vi "Get Weight.vi"(8 "error in (no error)":errorcluster caption="entrée d'erreur (pas d'erreur)", 11 "Class Balance_Adam_GBK en entrée":refnum<class "Class Balance_Adam_GBK.lvclass">) -> (0 "error out":errorcluster caption="sortie d'erreur", 2 "Get Weight":dbl, 3 "Class Balance_Adam_GBK en sortie":refnum<class "Class Balance_Adam_GBK.lvclass">)   [LabVIEW 2020, in "Library Instrument & Equipement.lvlib" / "Library Balance.lvlib" / "Class Balance_Adam_GBK.lvclass"]
uses:
  Class Balance_Adam_GBK.lvclass
  C:/Users/ngarcin/OneDrive - Altyor/Standard TB/Class/Balance/Balance (Default)/Class Balance (Default).lvclass
  Class Balance_Adam_GBK.lvclass/Class Balance_Adam_GBK.ctl
  Commun VI/Library Commun.lvlib
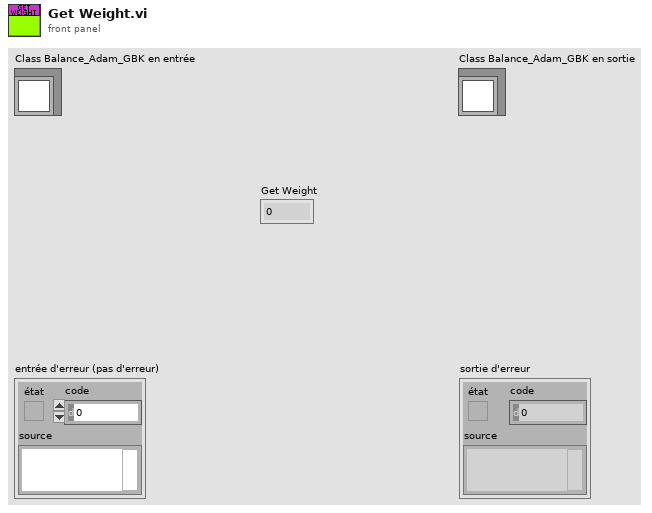
[diagram p1: front panel]
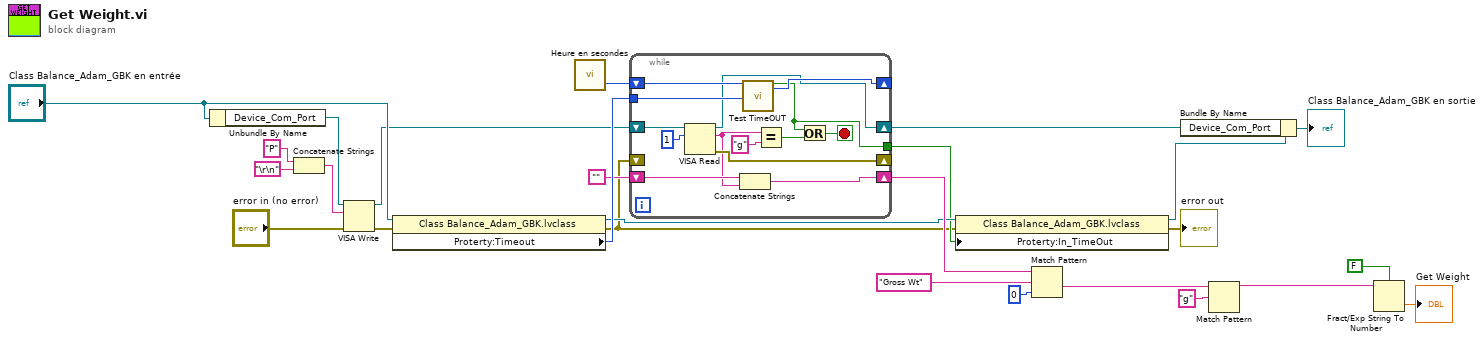
[diagram p0: block diagram]
diagram:
  n1 = Unbundle By Name("Class Balance_Adam_GBK en entrée") -> ("Device_Com_Port"=w22:refnum<visa-resource-name>)
  n2 = Concatenate Strings("P" ("chaîne"), "\r\n") -> (w25:string)
  n3 = VISA Write(VISA resource name=w22, write buffer=w25, error in (no error)="error in (no error)") -> (VISA resource name out=w17:refnum<visa-resource-name>, error out=w20:errorcluster)  [unwired: 1 out]
  n4 = property class="Class Balance_Adam_GBK.lvclass"(reference="Class Balance_Adam_GBK en entrée", error in=w20) -> (reference out=w5:refnum<class "Class Balance_Adam_GBK.lvclass">, error out=w1:errorcluster, "Proterty:Timeout"=w18:u32)
  n5 = call "Heure en secondes.vi"() -> ("Heure en milisecondes"=w21:u32)  [unwired: 2 in, 1 out]
  n6 = while {
    shift-right: [w39] -> _
    shift-left: w21 -> [w40]
    tunnel: w18 -> [w38]
    shift-right: [w34] -> w8
    shift-left: "" -> [w35]
    shift-right: [w33] -> _
    shift-left: w1 -> [_]
    shift-right: [w29] -> w15
    shift-left: w17 -> [w37]
    tunnel: [w27] -> w4
    stop <- w28 stop-if-true
    n7 = VISA Read(VISA resource name=w37, byte count=u32 1 ("nombre d'octets")) -> (VISA resource name out=w29:refnum<visa-resource-name>, read buffer=w32:string, error out=w33:errorcluster)  [unwired: 1 in, 1 out]
    n8 = Concatenate Strings(w35, w32) -> (w34:string)
    n9 = call "Test TimeOUT.vi"("OLD Time"=w40, "TimeOut ms"=w38) -> ("Timeout ?"=w27:bool, "NEW Time"=w39:u32)  [unwired: 13 in, 3 out]
    n10 = Equal?(x=w32, y="g") -> (x = y?=w30:bool)
    n11 = Or(x=w27, y=w30) -> (x .or. y?=w28:bool)
  }
  n12 = property class="Class Balance_Adam_GBK.lvclass"(reference=w5, error in=w1, "Proterty:In_TimeOut"=w4) -> (reference out=w3:refnum<class "Class Balance_Adam_GBK.lvclass">, error out=→"error out":errorcluster)
  n13 = Match Pattern(string=w8, regular expression="Gross Wt" ("expression régulière"), offset (0)=0) -> (after substring=w12:string)  [unwired: 3 out]
  n14 = Bundle By Name(cluster=w3, "Device_Com_Port"=w15) -> (→"Class Balance_Adam_GBK en sortie":refnum<class "Class Balance_Adam_GBK.lvclass">)
  n15 = Match Pattern(string=w12, regular expression="g" ("expression régulière")) -> (before substring=w10:string)  [unwired: 1 in, 3 out]
  n16 = Fract/Exp String To Number(use system decimal point (T)=FALSE ("utiliser le séparateur décimal du système (V)"), string=w10) -> (number=→"Get Weight":dbl)  [unwired: 2 in, 1 out]
